vi "Periodic Tasks.vi"(8 "error in":errorcluster) -> ()   [LabVIEW 2015]
doc: "This VI runs in parallel to other tasks. It can contain as many user-defined periodic loops as you need. These can carry out PID or other sorts of timed response."
uses:
  <vilib>/Rock Robotics/WPI/Solenoid/WPI_SolenoidValue.ctl
  Robot Global Data.vi
  <vilib>/Rock Robotics/Network Tables/NT Write Boolean.vi
  <vilib>/Rock Robotics/WPI/Solenoid/WPI_SolenoidSetEnum.vi
  <vilib>/Rock Robotics/WPI/Utilities/WPI_GetSetVariantRefNum.vi
  <vilib>/Rock Robotics/WPI/RobotDrive/WPI_RobotDriveArcadeDrive_Standard(NoSaturation).vi
  <vilib>/addons/control/pid/pid.llb/PID (DBL).vi
  <vilib>/Rock Robotics/Network Tables/NT Read Number.vi
  <vilib>/Rock Robotics/Network Tables/NT Read Numeric Array.vi
  <vilib>/addons/control/pid/NI_PID_pid.lvlib
panel:
  out "arm pot":dbl=0.28232946019173183
  in  "hanger":dbl
  in  "Cock":u32=2
  in  "Close intake":u32=2
  in  "Shot":u32=2
  in  "Intake":u32=2
  in  "lower limit":dbl=0.2
  in  "upper limit":dbl=0.4
  out "output":dbl=0.03019956748211805 format="%.2f"
  in  "PID gains":T1={"proportional gain (Kc)"=4.0, "integral time (Ti, min)"=0.0, "derivative time (Td, min)"=0.0} {"derivative time (Td, min)" format="%.3f"; "integral time (Ti, min)" format="%.3f"; "proportional gain (Kc)" format="%.3f"}
  in  "output range":cluster{"output high":dbl, "output low":dbl}={"output high"=0.4, "output low"=-0.4} {"output low" format="%.2f"; "output high" format="%.2f"}
  # "Shot Sequence Timing"
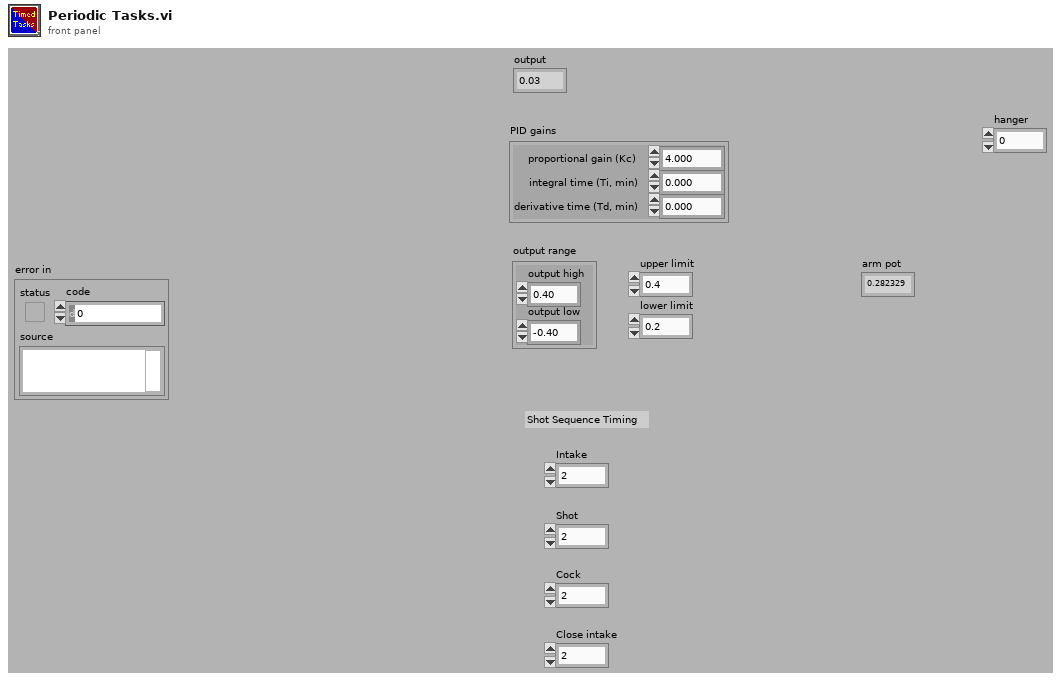
[diagram p1: front panel]
types:
  T1 = cluster{"proportional gain (Kc)":dbl, "integral time (Ti, min)":dbl, "derivative time (Td, min)":dbl}
  T2 = typedef "WPI_PotentiometerDevRef.ctl" = cluster{"DevStatus":errorcluster, "Analog Channel":T3, "Invert Output":bool}
  T3 = typedef "FPGA_AIChannel.ctl" = enum8{"AI 0", "AI 1", "AI 2", "AI 3", "AI MXP 0", "AI MXP 1", "AI MXP 2", "AI MXP 3", "Invalid"}
  T4 = typedef "WPI_EncoderDevRef.ctl" = cluster{"DevStatus":errorcluster, "EncoderIndex":T5, "CounterIndex":T6, "DistancePerCount":dbl, "Decoding Type":T7}
  T5 = typedef "FPGA_EncoderIdx.ctl" = enum8{"Enc 0", "Enc 1", "Enc 2", "Enc 3", "Enc 4", "Enc 5", "Enc 6", "Enc 7", "Invalid"}
  T6 = typedef "FPGA_CounterCtrSystemIndex.ctl" = enum8{"Ctr 0", "Ctr 1", "Ctr 2", "Ctr 3", "Ctr 4", "Ctr 5", "Ctr 6", "Ctr 7", "Invalid"}
  T7 = typedef "WPI_EncoderType.ctl" = enum16{"1x", "2x", "4x"}
  T8 = typedef "WPI_SolenoidDevRef.ctl" = cluster{"DevStatus":errorcluster, "Pneumatics Control Module":u8, "Forward Solenoid Channel":T9, "Reverse Solenoid Channel":T9}
  T9 = typedef "WPI_SolenoidChannel.ctl" = enum8{"Solenoid 0", "Solenoid 1", "Solenoid 2", "Solenoid 3", "Solenoid 4", "Solenoid 5", "Solenoid 6", "Solenoid 7", "Invalid"}
  T10 = typedef "WPI_RobotDriveDevRef.ctl" = cluster{"DevStatus":errorcluster, "Motors[]":T11[], "Square Inputs":bool, "Max Output":dbl}
  T11 = typedef "WPI_MotorControlDeviceRef.ctl" = cluster{"DeviceStatus":errorcluster, "Type":T12, "PWM":cluster{"PWM Channel":T13, "DeadBand":T14}, "CAN":cluster{"Device Number":u8, "Control Mode":T15, "Semaphore":T16, "Max Vout":dbl, "TalonSRX Control Mode":T17}, "Invert":bool}
  T12 = typedef "WPI_MotorControlType.ctl" = enum16{"PWM", "CAN", "CANTalonSRX"}
  T13 = typedef "FPGA_DIOPWMChannel.ctl" = enum8{"PWM 0", "PWM 1", "PWM 2", "PWM 3", "PWM 4", "PWM 5", "PWM 6", "PWM 7", "PWM 8", "PWM 9", "PWM MXP 0", "PWM MXP 1", "PWM MXP 2", "PWM MXP 3", "PWM MXP 4", "PWM MXP 5", "PWM MXP 6", "PWM MXP 7", "PWM MXP 8", "PWM MXP 9", "Invalid"}
  T14 = typedef "WPI_PWMDeadband.ctl" = cluster{"Name":string, "maxPositivePwm":i32, "minPositivePwm":i32, "centerPwm":i32, "maxNegativePwm":i32, "minNegativePwm":i32, "angularRange":u16}
  T15 = typedef "WPI_CANJaguar_ControlMode.ctl" = enum8{"Percent VBus", "Current", "Speed", "Position", "Voltage"}
  T16 = typedef "Semaphore RefNum" = refnum<k1>
  T17 = typedef "WPI_CANTalonSRX_APIControlMode.ctl" = enum8{"Percent VBus", "Speed", "Position", "Slave", "Unchanged / Invalid", "Voltage Compensation", "Current", "Motion Profile"}
  T18 = typedef "WPI_SolenoidValue.ctl" = enum16{"Off", "On", "Forward", "Reverse"}
  T19 = typedef "WPI_AnalogChannelDevRef.ctl" = cluster{"DevStatus":errorcluster, "Analog Channel":T3}
  T20 = cluster{"SolenoidDevRef":T8, "SolenoidDevRef":T8, "SolenoidDevRef":T8, "SolenoidDevRef":T8, "SolenoidDevRef":T8}
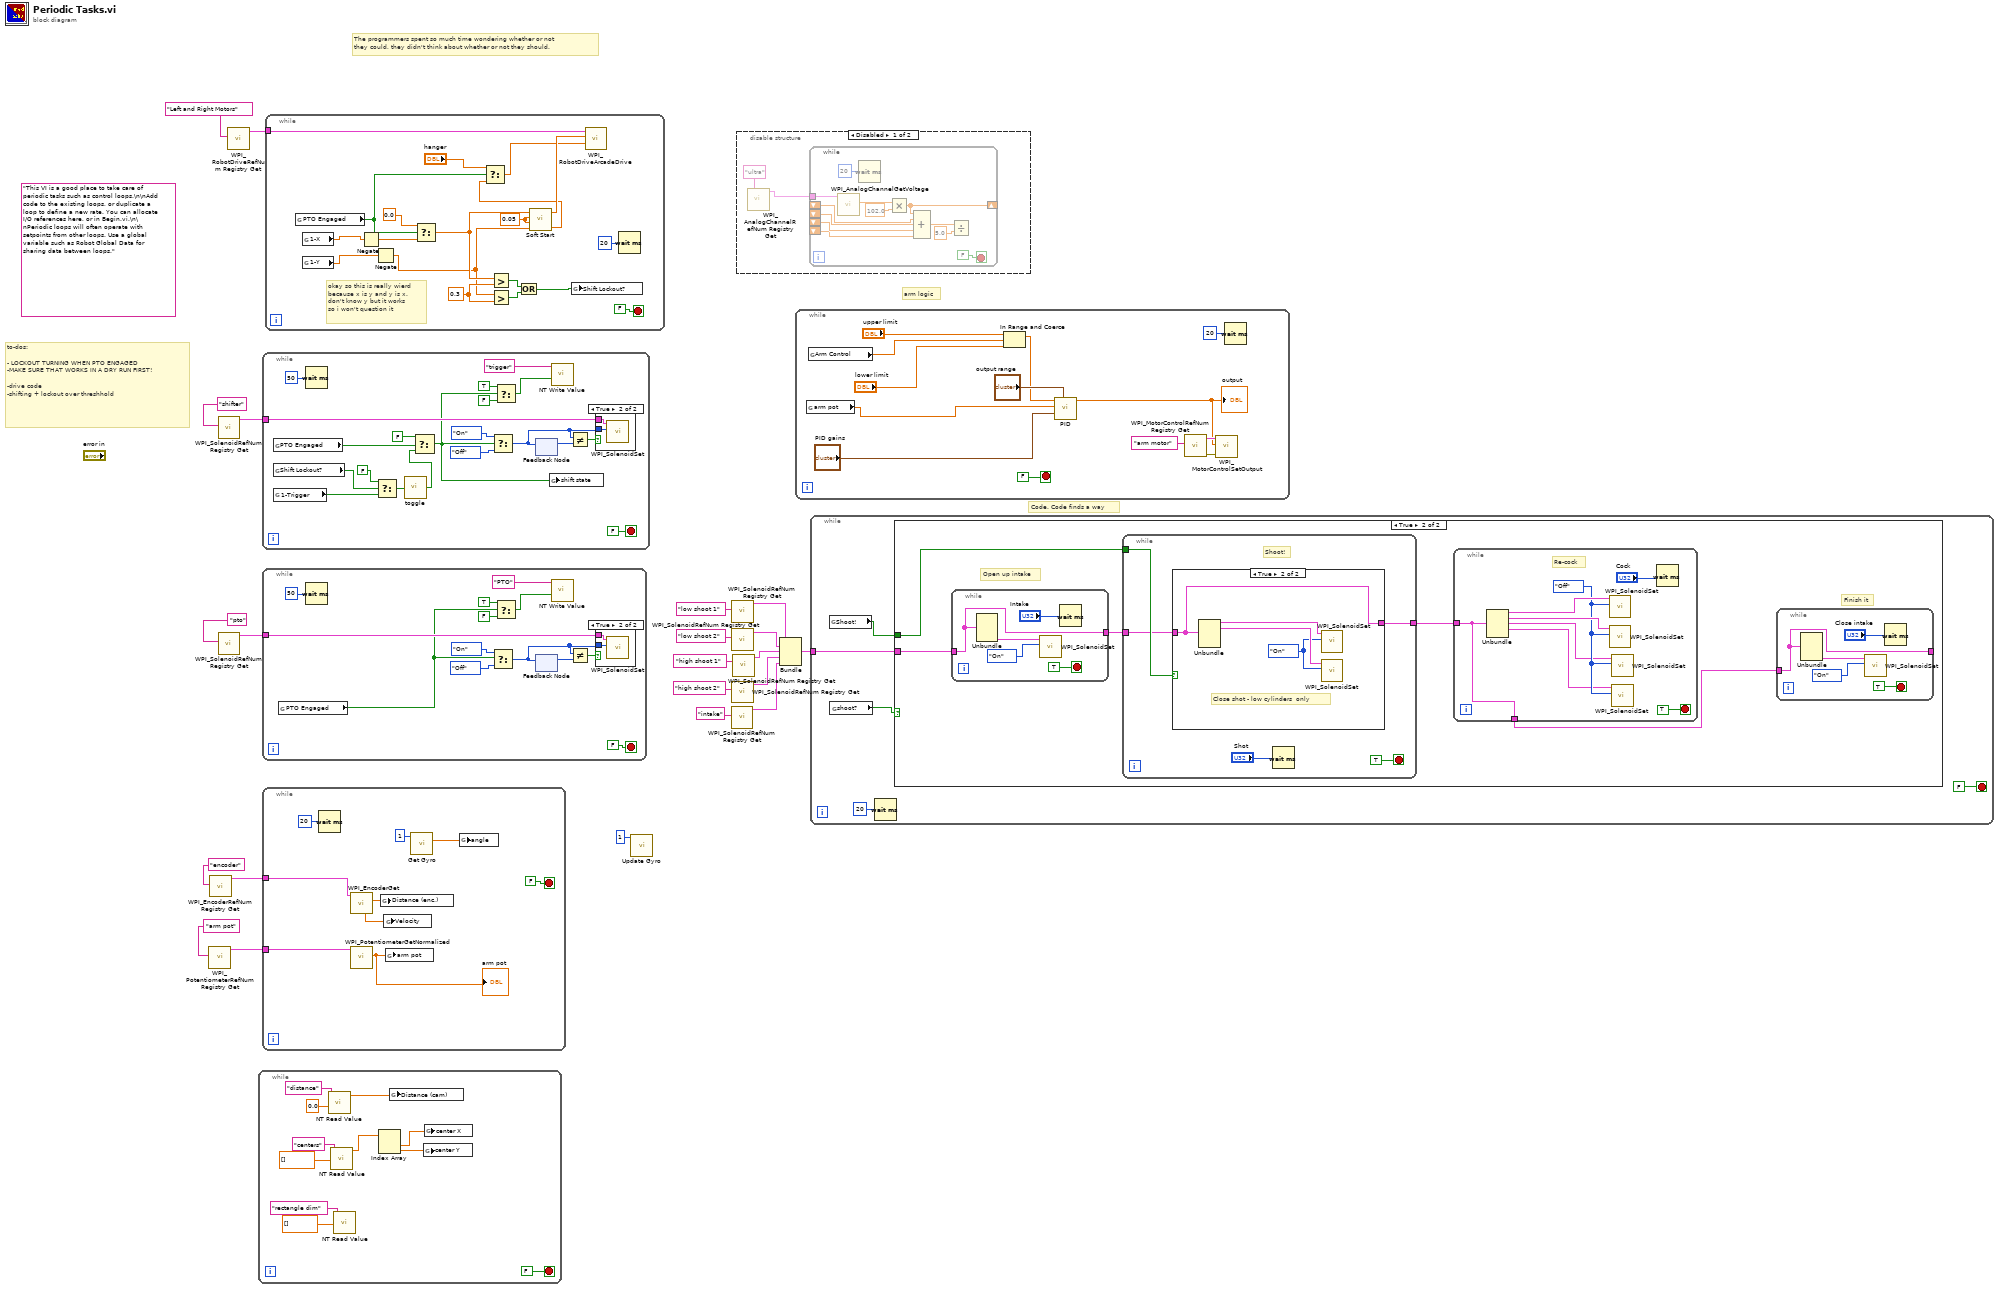
[diagram p0: block diagram]
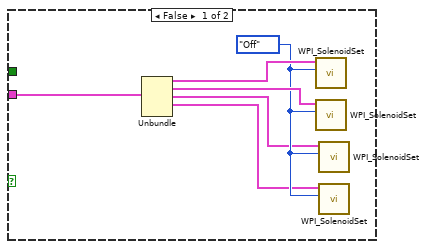
[diagram p3: hidden frame]
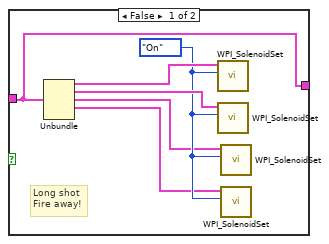
[diagram p4: hidden frame]
diagram:
  (unwired) "This VI is a good place to take care of periodic tasks such as control loops.\n\nAdd code to the existing loops, or duplicate a loop to define a new rate. You can allocate I/O references here, or in Begin.vi.\n\nPeriodic loops will often operate with setpoints from other loops. Use a global variable such as Robot Global Data for sharing data between loops."
  # "arm logic"
  # "The programmers spent so much time wondering whether or not\nthey could, they didn't think about whether or not they should."
  # "Code. Code finds a way"
  # "to-dos:\n\n- LOCKOUT TURNING WHEN PTO ENGAGED\n-MAKE SURE THAT WORKS IN A DRY RUN FIRST!\n\n-drive code\n-shifting + lockout over threshhold"
  n1 = call <vilib>:"WPI_PotentiometerRefNum Registry Get.vi"("refnum name"="arm pot") -> ("PotDevRef"=w13:T2)  [unwired: 9 in, 1 out]
  n2 = call <vilib>:"WPI_EncoderRefNum Registry Get.vi"("refnum name"="encoder") -> ("EncoderDevRef"=w17:T4)  [unwired: 9 in, 1 out]
  n3 = call <vilib>:"WPI_SolenoidRefNum Registry Get.vi"("refnum name"="shifter") -> ("SolenoidDevRef"=w21:T8)  [unwired: 9 in, 1 out]
  n4 = call <vilib>:"WPI_SolenoidRefNum Registry Get.vi"("refnum name"="pto") -> ("SolenoidDevRef"=w15:T8)  [unwired: 9 in, 1 out]
  n5 = call <vilib>:"WPI_RobotDriveRefNum Registry Get.vi"("refnum name"="Left and Right Motors") -> ("RobotDriveDevRef"=w19:T10)  [unwired: 9 in, 1 out]
  n6 = while {
    stop <- FALSE stop-if-true
    n7 = call-poly <vilib>:"NT Read Value.vi"("Default Value"=0.0, "Name"="distance") -> ("Numeric"=w26:dbl)  [unwired: 8 in, 1 out]
    n8 = call-poly <vilib>:"NT Read Value.vi"("Default Value"=dbl[] [], "Name"="centers") -> ("Numeric Array"=w25:dbl[])  [unwired: 8 in, 1 out]
    n9 = call-poly <vilib>:"NT Read Value.vi"("Default Value"=dbl[] [], "Name"="rectangle dim") -> ()  [unwired: 8 in, 2 out]
    n10 = Index Array(array=w25) -> (element #1=w24:dbl, element #2=w23:dbl)  [unwired: 2 in]
    n11 = global write "Robot Global Data.vi" "Distance (cam)"(w26) -> ()
    n12 = global write "Robot Global Data.vi" "center Y"(w23) -> ()
    n13 = global write "Robot Global Data.vi" "center X"(w24) -> ()
  }
  n14 = while {
    tunnel: w21 -> [w40]
    stop <- FALSE stop-if-true
    n15 = global read "Robot Global Data.vi" "PTO Engaged"() -> (w38:bool)
    n16 = global read "Robot Global Data.vi" "Shift Lockout?"() -> (w42:bool)
    n17 = global read "Robot Global Data.vi" "1-Trigger"() -> (w43:bool)
    n18 = Wait (ms)(milliseconds to wait=u32 50) -> ()  [unwired: 1 out]
    n19 = Select(t=FALSE, s=w42, f=w43) -> (s? t:f=w39:bool)
    n20 = call "toggle.vi"("Input"=w39) -> ("Output"=w37:bool)
    n21 = Select(t=FALSE, s=w38, f=w37) -> (s? t:f=w34:bool)
    n22 = Select(t=WPI_SolenoidValue."On" ("Value"), s=w34, f=WPI_SolenoidValue."Off" ("Value")) -> (s? t:f=w35:T18)
    n23 = Select(t=TRUE, s=w34, f=FALSE) -> (s? t:f=w48:bool)
    n24 = feedback #1() -> (w44:T18)  [unwired: 1 in]
    n25 = feedback-in #1(w35) -> ()
    n26 = global write "Robot Global Data.vi" "shift state"(w34) -> ()
    n27 = call-poly <vilib>:"NT Write Value.vi"("Boolean"=w48, "Name"="trigger") -> ()  [unwired: 9 in, 1 out]
    n28 = Not Equal?(x=w35, y=w44) -> (x != y?=w45:bool)
    n29 = case shown="True" w45 {
      tunnel: w35 -> [_ w55]
      tunnel: w40 -> [_ w54]
      frame False {
      }
      frame True {
        n30 = call-poly <vilib>:"WPI_SolenoidSet.vi"("Value"=w55, "SolenoidDevRef"=w54) -> ()  [unwired: 8 in, 2 out]
      }
    }
  }
  n31 = while {
    tunnel: w15 -> [w57]
    stop <- FALSE stop-if-true
    n32 = global read "Robot Global Data.vi" "PTO Engaged"() -> (w56:bool)
    n33 = Wait (ms)(milliseconds to wait=u32 50) -> ()  [unwired: 1 out]
    n34 = Select(t=WPI_SolenoidValue."On" ("Value"), s=w56, f=WPI_SolenoidValue."Off" ("Value")) -> (s? t:f=w58:T18)
    n35 = Select(t=TRUE, s=w56, f=FALSE) -> (s? t:f=w63:bool)
    n36 = feedback #2() -> (w59:T18)  [unwired: 1 in]
    n37 = feedback-in #2(w58) -> ()
    n38 = call-poly <vilib>:"NT Write Value.vi"("Boolean"=w63, "Name"="PTO") -> ()  [unwired: 9 in, 1 out]
    n39 = Not Equal?(x=w58, y=w59) -> (x != y?=w60:bool)
    n40 = case shown="True" w60 {
      tunnel: w58 -> [_ w70]
      tunnel: w57 -> [_ w69]
      frame False {
      }
      frame True {
        n41 = call-poly <vilib>:"WPI_SolenoidSet.vi"("Value"=w70, "SolenoidDevRef"=w69) -> ()  [unwired: 8 in, 2 out]
      }
    }
  }
  n42 = while {
    tunnel: w17 -> [w75]
    tunnel: w13 -> [w74]
    stop <- FALSE stop-if-true
    n43 = Wait (ms)(milliseconds to wait=u32 20) -> ()  [unwired: 1 out]
    n44 = call <vilib>:"WPI_EncoderGet.vi"("EncoderDevRef"=w75) -> ("Distance"=w77:dbl, "Rate"=w76:dbl)  [unwired: 5 in, 4 out]
    n45 = call <vilib>:"WPI_PotentiometerGetNormalized.vi"("PotDevRef"=w74) -> ("Normalized Value"=w71:dbl)  [unwired: 8 in, 2 out]
    "arm pot" <- w71
    n46 = global write "Robot Global Data.vi" "Distance (enc.)"(w77) -> ()
    n47 = global write "Robot Global Data.vi" "Velocity"(w76) -> ()
    n48 = global write "Robot Global Data.vi" "arm pot"(w71) -> ()
    n49 = call "Get Gyro.vi"("Gyro ID (1 or 2)"=1) -> ("Angle"=w72:dbl)  [unwired: 9 in, 1 out]
    n50 = global write "Robot Global Data.vi" "angle"(w72) -> ()
  }
  n51 = while {
    tunnel: w19 -> [w96]
    stop <- FALSE stop-if-true
    w88 = 0.05 ("X-Slew Rate")
    w91 = 0.3 ("y")
    # "okay so this is really wierd\nbecause x is y and y is x.\ndon't know y but it works \nso i won't question it"
    n52 = global read "Robot Global Data.vi" "PTO Engaged"() -> (w85:bool)
    n53 = global read "Robot Global Data.vi" "1-X"() -> (w81:dbl)
    n54 = global read "Robot Global Data.vi" "1-Y"() -> (w80:dbl)
    n55 = Negate(x=w81) -> (-x=w83:dbl)
    n56 = Negate(x=w80) -> (-x=w82:dbl)
    n57 = Select(t=0.0, s=w85, f=w83) -> (s? t:f=w90:dbl)
    n58 = Greater?(x=w82, y=w91) -> (0:w94:bool)
    n59 = Greater?(x=w90, y=w91) -> (0:w92:bool)
    n60 = Or(x=w92, y=w94) -> (x .or. y?=w93:bool)
    n61 = call "Soft Start.vi"("X- axis Joystick"=w90, "X-Slew Rate"=w88, "Y-Slew Rate"=w88, "Y-axis Joystick"=w82) -> ("X-axis drive"=w89:dbl, "Y-axis drive"=w86:dbl)  [unwired: 2 in, 1 out]
    n62 = Select(t="hanger", s=w85, f=w86) -> (s? t:f=w87:dbl)
    n63 = global write "Robot Global Data.vi" "Shift Lockout?"(w93) -> ()
    n64 = call-poly <vilib>:"WPI_RobotDriveArcadeDrive.vi"("Y axis value"=w87, "X axis value"=w89, "RobotDriveDevRef"=w96) -> ()  [unwired: 6 in, 3 out]
    n65 = Wait (ms)(milliseconds to wait=u32 20) -> ()  [unwired: 1 out]
  }
  n66 = call "Update Gyro.vi"("Gyro ID (1 or 2)"=1) -> ()  [unwired: 11 in]
  n67 = call <vilib>:"WPI_SolenoidRefNum Registry Get.vi"("refnum name"="intake") -> ("SolenoidDevRef"=w7:T8)  [unwired: 9 in, 1 out]
  n68 = call <vilib>:"WPI_SolenoidRefNum Registry Get.vi"("refnum name"="low shoot 1") -> ("SolenoidDevRef"=w3:T8)  [unwired: 9 in, 1 out]
  n69 = call <vilib>:"WPI_SolenoidRefNum Registry Get.vi"("refnum name"="low shoot 2") -> ("SolenoidDevRef"=w4:T8)  [unwired: 9 in, 1 out]
  n70 = call <vilib>:"WPI_SolenoidRefNum Registry Get.vi"("refnum name"="high shoot 2") -> ("SolenoidDevRef"=w6:T8)  [unwired: 9 in, 1 out]
  n71 = call <vilib>:"WPI_SolenoidRefNum Registry Get.vi"("refnum name"="high shoot 1") -> ("SolenoidDevRef"=w5:T8)  [unwired: 9 in, 1 out]
  n72 = disable-structure shown="Disabled" {
    frame Disabled {
      n73 = call <vilib>:"WPI_AnalogChannelRefNum Registry Get.vi"("refnum name"="ultra") -> ("AIDeviceRef"=w99:T19)  [unwired: 9 in, 1 out]
      n74 = while {
        shift-right: [w108] -> _
        shift-left: _ -> [w107]
        shift-left: _ -> [w106]
        shift-left: _ -> [w105]
        shift-left: _ -> [w104]
        tunnel: w99 -> [w101]
        stop <- FALSE stop-if-true
        n75 = call <vilib>:"WPI_AnalogChannelGetVoltage.vi"("AIDeviceRef"=w101) -> ("Voltage"=w109:dbl)  [unwired: 8 in, 2 out]
        n76 = Wait (ms)(milliseconds to wait=u32 20) -> ()  [unwired: 1 out]
        n77 = Multiply(x=w109, y=102.0) -> (x*y=w108:dbl)
        n78 = Compound Arithmetic op=ADD(w108, w107, w106, w105, w104) -> (w103:dbl)
        n79 = Divide(x=w103, y=5.0) -> ()  [unwired: 1 out]
      }
    }
    frame Enabled {
    }
  }
  n80 = Bundle("SolenoidDevRef"=w3, "SolenoidDevRef"=w4, "SolenoidDevRef"=w5, "SolenoidDevRef"=w6, "SolenoidDevRef"=w7) -> (w2:T20)  [unwired: 1 in]
  n81 = while {
    stop <- FALSE stop-if-true
    n82 = global read "Robot Global Data.vi" "arm pot"() -> (w113:dbl)
    n83 = global read "Robot Global Data.vi" "Arm Control"() -> (w120:dbl)
    n84 = In Range and Coerce(upper limit="upper limit", x=w120, lower limit="lower limit") -> (coerced(x)=w119:dbl)  [unwired: 1 out]
    n85 = call-poly <vilib>:"PID.vi"("output range"="output range", "PID gains"="PID gains", "process variable"=w113, "setpoint"=w119) -> ("output"=w114:dbl)  [unwired: 6 in, 1 out]
    "output" <- w114
    n86 = call <vilib>:"WPI_MotorControlRefNum Registry Get.vi"("refnum name"="arm motor") -> ("error out"=w116:errorcluster, "MotorControlDevRef"=w115:T11)  [unwired: 9 in]
    n87 = call <vilib>:"WPI_MotorControlSetOutput.vi"("error in (no error)"=w116, "Output"=w114, "MotorControlDevRef"=w115) -> ()  [unwired: 6 in, 3 out]
    n88 = Wait (ms)(milliseconds to wait=u32 20) -> ()  [unwired: 1 out]
  }
  n89 = while {
    tunnel: w2 -> [w130]
    stop <- FALSE stop-if-true
    n90 = global read "Robot Global Data.vi" "Shoot!"() -> (w129:bool)
    n91 = global read "Robot Global Data.vi" "shoot?"() -> (w126:bool)
    n92 = Wait (ms)(milliseconds to wait=u32 20) -> ()  [unwired: 1 out]
    n93 = case shown="True" w126 {
      tunnel: w130 -> [w131 w141]
      tunnel: w129 -> [_ w140]
      frame False {
        w134 = WPI_SolenoidValue."Off" ("Value")
        n94 = Unbundle(w131) -> ("SolenoidDevRef"=w136:T8, "SolenoidDevRef"=w135:T8, "SolenoidDevRef"=w133:T8, "SolenoidDevRef"=w132:T8)  [unwired: 1 out]
        n95 = call-poly <vilib>:"WPI_SolenoidSet.vi"("Value"=w134, "SolenoidDevRef"=w136) -> ()  [unwired: 8 in, 2 out]
        n96 = call-poly <vilib>:"WPI_SolenoidSet.vi"("Value"=w134, "SolenoidDevRef"=w135) -> ()  [unwired: 8 in, 2 out]
        n97 = call-poly <vilib>:"WPI_SolenoidSet.vi"("Value"=w134, "SolenoidDevRef"=w133) -> ()  [unwired: 8 in, 2 out]
        n98 = call-poly <vilib>:"WPI_SolenoidSet.vi"("Value"=w134, "SolenoidDevRef"=w132) -> ()  [unwired: 8 in, 2 out]
      }
      frame True {
        # "Finish it"
        # "Open up intake"
        n99 = while {
          tunnel: w141 -> [w170]
          tunnel: [w170] -> w139
          stop <- TRUE stop-if-true
          n100 = Unbundle(w170) -> ("SolenoidDevRef"=w171:T8)  [unwired: 4 out]
          n101 = call-poly <vilib>:"WPI_SolenoidSet.vi"("Value"=WPI_SolenoidValue."On", "SolenoidDevRef"=w171) -> ()  [unwired: 8 in, 2 out]
          n102 = Wait (ms)(milliseconds to wait="Intake") -> ()  [unwired: 1 out]
        }
        n103 = while {
          tunnel: w140 -> [w159]
          tunnel: w139 -> [w156]
          tunnel: [w155] -> w138
          stop <- TRUE stop-if-true
          # "Shoot!"
          n104 = case shown="True" w159 {
            tunnel: w156 -> [w160 w166]
            tunnel: [w160 w166] -> w155
            frame False {
              w163 = WPI_SolenoidValue."On" ("Value")
              # "Long shot\nFire away!"
              n105 = Unbundle(w160) -> ("SolenoidDevRef"=w165:T8, "SolenoidDevRef"=w164:T8, "SolenoidDevRef"=w162:T8, "SolenoidDevRef"=w161:T8)  [unwired: 1 out]
              n106 = call-poly <vilib>:"WPI_SolenoidSet.vi"("Value"=w163, "SolenoidDevRef"=w165) -> ()  [unwired: 8 in, 2 out]
              n107 = call-poly <vilib>:"WPI_SolenoidSet.vi"("Value"=w163, "SolenoidDevRef"=w164) -> ()  [unwired: 8 in, 2 out]
              n108 = call-poly <vilib>:"WPI_SolenoidSet.vi"("Value"=w163, "SolenoidDevRef"=w162) -> ()  [unwired: 8 in, 2 out]
              n109 = call-poly <vilib>:"WPI_SolenoidSet.vi"("Value"=w163, "SolenoidDevRef"=w161) -> ()  [unwired: 8 in, 2 out]
            }
            frame True {
              w167 = WPI_SolenoidValue."On" ("Value")
              # "Close shot - low cylinders  only"
              n110 = Unbundle(w166) -> ("SolenoidDevRef"=w169:T8, "SolenoidDevRef"=w168:T8)  [unwired: 3 out]
              n111 = call-poly <vilib>:"WPI_SolenoidSet.vi"("Value"=w167, "SolenoidDevRef"=w169) -> ()  [unwired: 8 in, 2 out]
              n112 = call-poly <vilib>:"WPI_SolenoidSet.vi"("Value"=w167, "SolenoidDevRef"=w168) -> ()  [unwired: 8 in, 2 out]
            }
          }
          n113 = Wait (ms)(milliseconds to wait="Shot") -> ()  [unwired: 1 out]
        }
        n114 = while {
          tunnel: w138 -> [w148]
          tunnel: [w148] -> w137
          stop <- TRUE stop-if-true
          w152 = WPI_SolenoidValue."Off" ("Value")
          # "Re-cock"
          n115 = Unbundle(w148) -> ("SolenoidDevRef"=w154:T8, "SolenoidDevRef"=w153:T8, "SolenoidDevRef"=w151:T8, "SolenoidDevRef"=w150:T8)  [unwired: 1 out]
          n116 = call-poly <vilib>:"WPI_SolenoidSet.vi"("Value"=w152, "SolenoidDevRef"=w154) -> ()  [unwired: 8 in, 2 out]
          n117 = call-poly <vilib>:"WPI_SolenoidSet.vi"("Value"=w152, "SolenoidDevRef"=w153) -> ()  [unwired: 8 in, 2 out]
          n118 = call-poly <vilib>:"WPI_SolenoidSet.vi"("Value"=w152, "SolenoidDevRef"=w151) -> ()  [unwired: 8 in, 2 out]
          n119 = call-poly <vilib>:"WPI_SolenoidSet.vi"("Value"=w152, "SolenoidDevRef"=w150) -> ()  [unwired: 8 in, 2 out]
          n120 = Wait (ms)(milliseconds to wait="Cock") -> ()  [unwired: 1 out]
        }
        n121 = while {
          tunnel: w137 -> [w142]
          tunnel: [w142] -> _
          stop <- TRUE stop-if-true
          n122 = Unbundle(w142) -> ("SolenoidDevRef"=w143:T8)  [unwired: 4 out]
          n123 = call-poly <vilib>:"WPI_SolenoidSet.vi"("Value"=WPI_SolenoidValue."On", "SolenoidDevRef"=w143) -> ()  [unwired: 8 in, 2 out]
          n124 = Wait (ms)(milliseconds to wait="Close intake") -> ()  [unwired: 1 out]
        }
      }
    }
  }
